vi "shooter_state_machine.vi"() -> ()   [LabVIEW 2013]
panel:
  out "Large_Cylinder_Med_Timer":i32=2000
  in  "Arm_Shooter_High":bool
  out "LAST_Shooter_Command":string
  in  "Aim":bool
  in  "Shoot":bool
  in  "Arm_Shooter_Medium":bool
  out "LAST_SHOOTER_STATE":string
  in  "Rest_Shooter":bool
  out "Large_Cylinder_CMD":bool
  out "Small_Cylinder_CMD":bool
  out "Small_Cylinder_Timer":i32=1000
  out "Large_Cylinder_High_Timer":i32=4000
  out "Shooter_Command":string
  out "Small_Cylinder_State":u8(slide) scale=0.0..1.0
  out "Large_Cylinder_State":u8(slide) scale=0.0..2.0
  out "SHOOTER_STATE":string
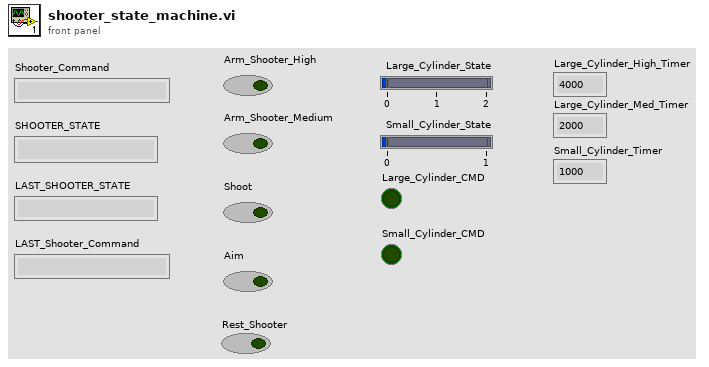
[diagram p1: front panel]
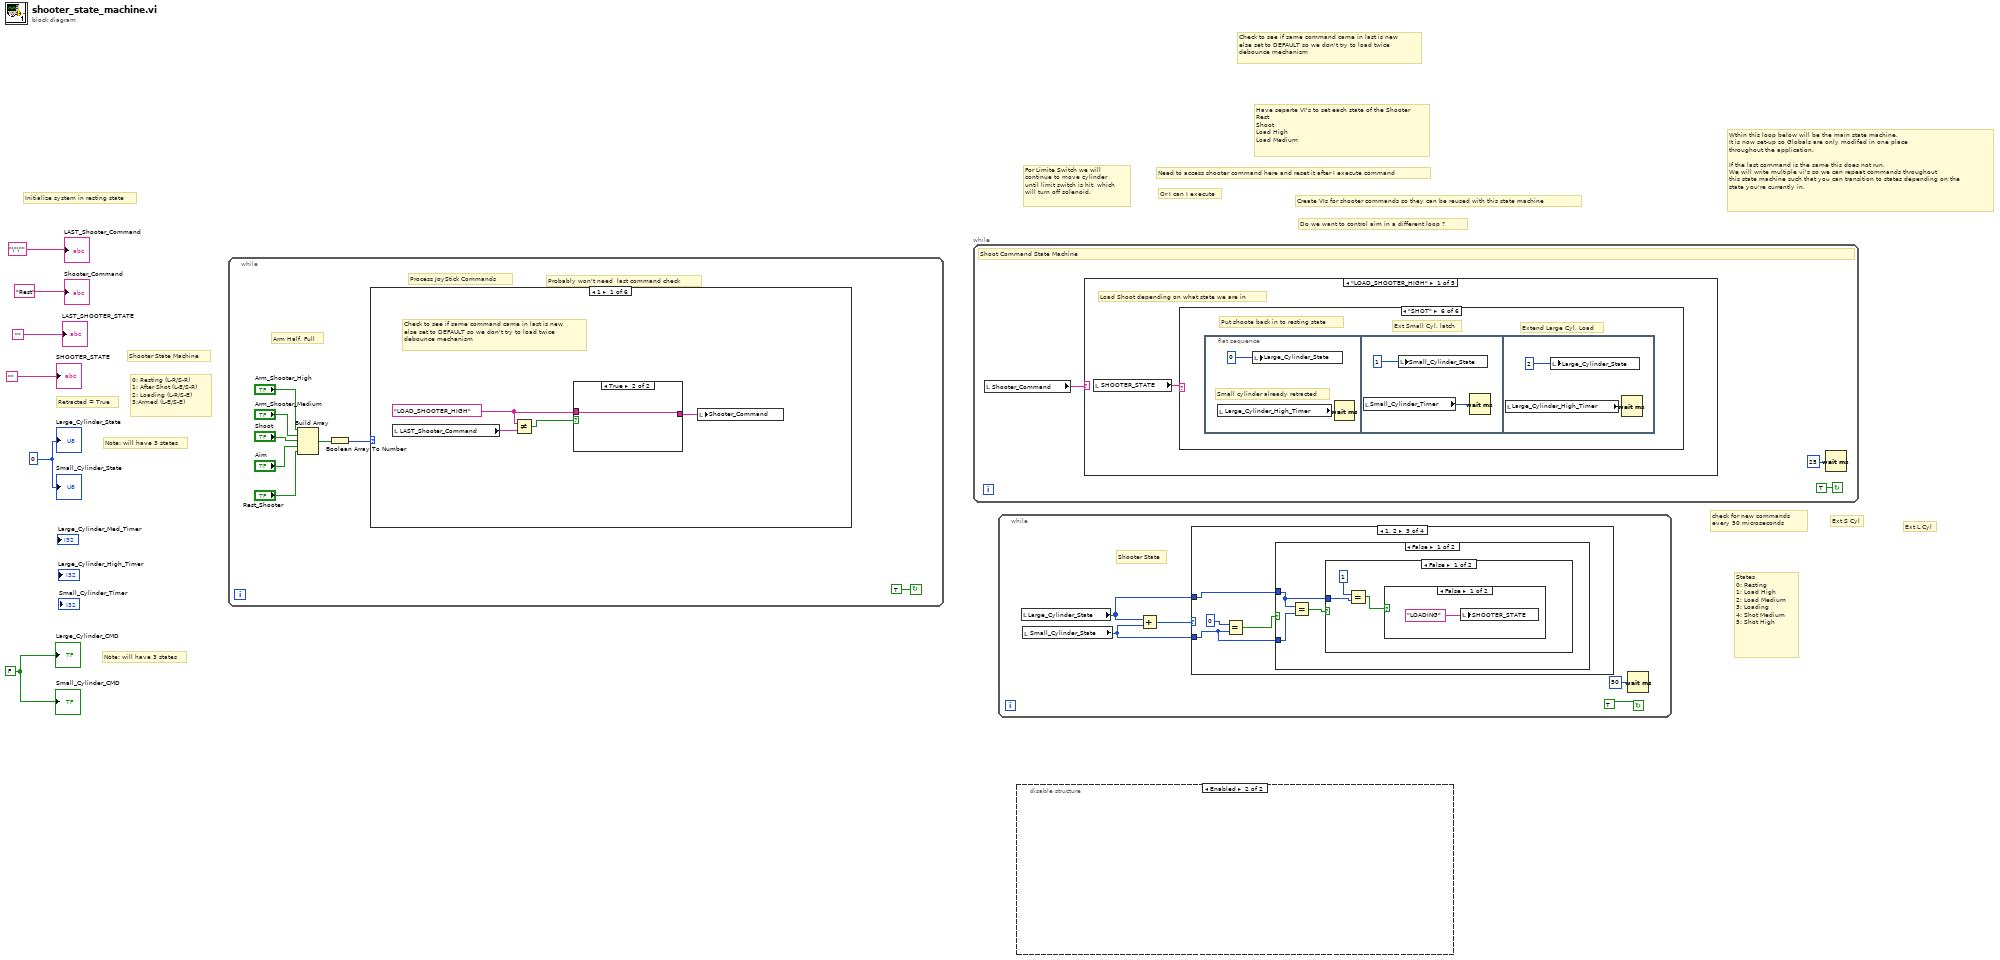
[diagram p0: block diagram]
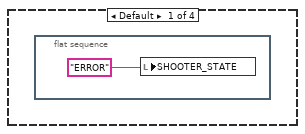
[diagram p2: hidden frame]
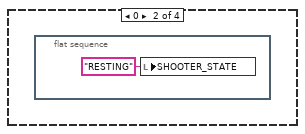
[diagram p3: hidden frame]
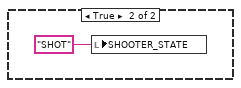
[diagram p4: hidden frame]
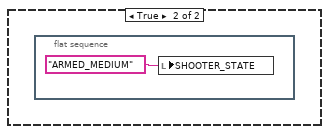
[diagram p5: hidden frame]
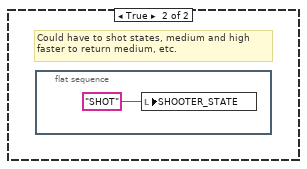
[diagram p6: hidden frame]
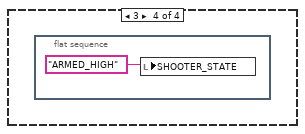
[diagram p7: hidden frame]
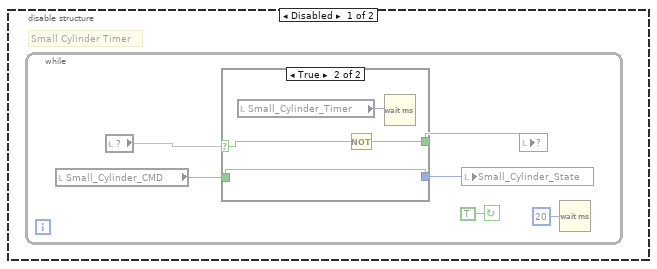
[diagram p8: hidden frame]
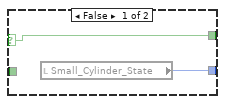
[diagram p9: hidden frame]
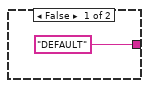
[diagram p10: hidden frame]
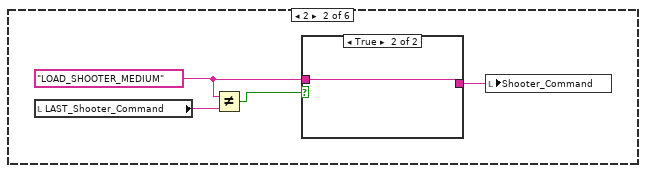
[diagram p11: hidden frame]
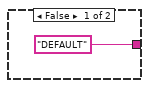
[diagram p12: hidden frame]
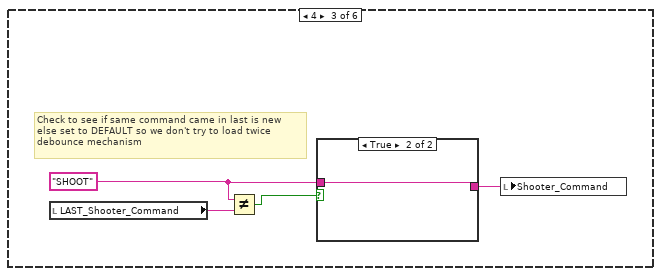
[diagram p13: hidden frame]
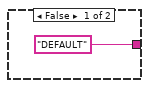
[diagram p14: hidden frame]
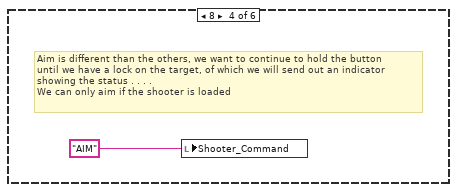
[diagram p15: hidden frame]
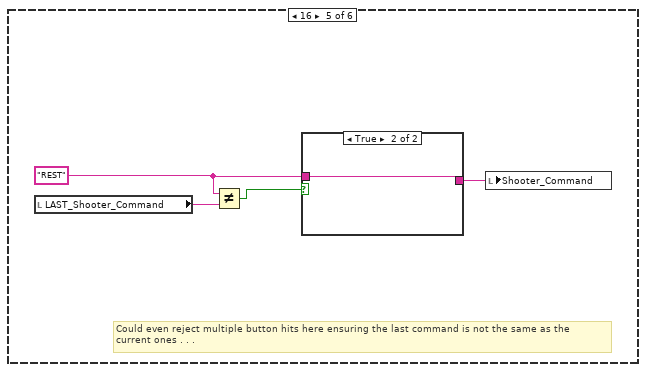
[diagram p16: hidden frame]
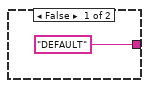
[diagram p17: hidden frame]
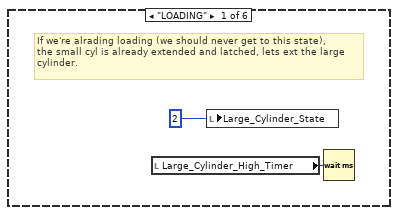
[diagram p19: hidden frame]
diagram:
  w1 = 0
  w4 = FALSE
  # "Do we want to control aim in a different loop ?"
  # "Ext L Cyl"
  # "Ext S Cyl"
  # "States\n0: Resting\n1: Load High\n2: Load Medium\n3: Loading\n4: Shot Medium\n5: Shot High"
  # "Have separte VI's to set each state of the Shooter\nRest\nShoot\nLoad High\nLoad Medium"
  # "Check to see if same command came in last is new\nelse set to DEFAULT so we don't try to load twice\ndebounce mechanism"
  # "Wthin this loop below will be the main state machine. \nIt is now set-up so Globals are only modifed in one place \nthroughout the application. \n\nIf the last command is the same this does not run.\nWe will write multiple vi's so we can repeat commands throughout\nthis state machine such that you can transition to states depending on the\nstate you're currently in."
  # "Create VIs for shooter commands so they can be reused with this state machine"
  # "check for new commands \nevery 50 microseconds"
  # "Or I can I execute"
  # "Need to access shooter command here and reset it after I execute command"
  # "Initialize system in resting state"
  # "Note: will have 3 states"
  # "0: Resting (L-R/S-R)\n1: After Shot (L-E/S-R)\n2: Loading (L-R/S-E)\n3:Armed (L-E/S-E)"
  # "For Limite Switch we will\ncontinue to move cylinder\nuntil limit switch is hit, which\nwill turn off solenoid."
  # "Note: will have 3 states"
  # "Shooter State Machine"
  # "Retracted = True"
  n1 = while {
    stop <- TRUE continue-if-true
    # "Probably won't need  last command check"
    # "Arm Half, Full"
    # "Process JoyStick Commands"
    n2 = Build Array("Arm_Shooter_High", "Arm_Shooter_Medium", "Shoot", "Aim", "Rest_Shooter") -> (w12:bool[])
    n3 = Boolean Array To Number(Boolean array=w12) -> (number=w13:u32)
    n4 = case shown="1" w13 {
      frame 1 {
        w16 = "LOAD_SHOOTER_HIGH"
        # "Check to see if same command came in last is new\nelse set to DEFAULT so we don't try to load twice\ndebounce mechanism"
        n5 = local read "LAST_Shooter_Command"() -> (w18:string)
        n6 = Not Equal?(x=w16, y=w18) -> (x != y?=w17:bool)
        n7 = case shown="True" w17 {
          tunnel: w16 -> [_ w20]
          tunnel: ["DEFAULT" w20] -> w15
          frame False {
          }
          frame True {
          }
        }
        n8 = local write "Shooter_Command"(w15) -> ()
      }
      frame 2 {
        w22 = "LOAD_SHOOTER_MEDIUM"
        n9 = local read "LAST_Shooter_Command"() -> (w24:string)
        n10 = Not Equal?(x=w22, y=w24) -> (x != y?=w23:bool)
        n11 = case shown="True" w23 {
          tunnel: w22 -> [_ w26]
          tunnel: ["DEFAULT" w26] -> w21
          frame False {
          }
          frame True {
          }
        }
        n12 = local write "Shooter_Command"(w21) -> ()
      }
      frame 4 {
        w28 = "SHOOT"
        # "Check to see if same command came in last is new\nelse set to DEFAULT so we don't try to load twice\ndebounce mechanism"
        n13 = local read "LAST_Shooter_Command"() -> (w30:string)
        n14 = Not Equal?(x=w28, y=w30) -> (x != y?=w29:bool)
        n15 = case shown="True" w29 {
          tunnel: w28 -> [_ w32]
          tunnel: ["DEFAULT" w32] -> w27
          frame False {
          }
          frame True {
          }
        }
        n16 = local write "Shooter_Command"(w27) -> ()
      }
      frame 8 {
        # "Aim is different than the others, we want to continue to hold the button\nuntil we have a lock on the target, of which we will send out an indicator \nshowing the status . . . . \nWe can only aim if the shooter is loaded"
        n17 = local write "Shooter_Command"("AIM") -> ()
      }
      frame 16 {
        w35 = "REST"
        # "Could even reject multiple button hits here ensuring the last command is not the same as the \ncurrent ones . . ."
        n18 = local read "LAST_Shooter_Command"() -> (w37:string)
        n19 = Not Equal?(x=w35, y=w37) -> (x != y?=w36:bool)
        n20 = case shown="True" w36 {
          tunnel: w35 -> [_ w39]
          tunnel: ["DEFAULT" w39] -> w34
          frame False {
          }
          frame True {
          }
        }
        n21 = local write "Shooter_Command"(w34) -> ()
      }
      frame Default {
        # "Do Nothing"
      }
    }
  }
  n22 = while "Shoot Command State Machine" {
    stop <- TRUE continue-if-true
    # "Shoot Command State Machine"
    n23 = local read "Shooter_Command"() -> (w40:string)
    n24 = case shown="\"LOAD_SHOOTER_HIGH\"" w40 {
      frame "LOAD_SHOOTER_HIGH" {
        # "Load Shoot depending on what state we are in"
        n25 = local read "SHOOTER_STATE"() -> (w43:string)
        n26 = case shown="\"SHOT\"" w43 {
          frame "LOADING" {
            # "If we're alrading loading (we should never get to this state), \nthe small cyl is already extended and latched, lets ext the large\ncylinder."
            n27 = local read "Large_Cylinder_High_Timer"() -> (w44:i32)
            n28 = local write "Large_Cylinder_State"(2) -> ()
            n29 = Wait (ms)(milliseconds to wait=w44) -> ()  [unwired: 1 out]
          }
          frame Default {
            # "Some kind of error state, should never find ourselves here"
          }
          frame "RESTING" {
            # "Ext L Cyl"
            # "Ext S Cyl"
            n30 = flat-sequence {
              frame #0 {
                n31 = local read "Small_Cylinder_Timer"() -> (w47:i32)
                n32 = local write "Small_Cylinder_State"(1) -> ()
                n33 = Wait (ms)(milliseconds to wait=w47) -> ()  [unwired: 1 out]
              }
              frame #1 {
                n34 = local read "Large_Cylinder_High_Timer"() -> (w48:i32)
                n35 = local write "Large_Cylinder_State"(2) -> ()
                n36 = Wait (ms)(milliseconds to wait=w48) -> ()  [unwired: 1 out]
              }
            }
          }
          frame "ARMED_MEDIUM" {
            # "Just need extend for half time"
            n37 = local write "Large_Cylinder_State"(2) -> ()
            n38 = local read "Large_Cylinder_Med_Timer"() -> (w50:i32)
            n39 = Wait (ms)(milliseconds to wait=w50) -> ()  [unwired: 1 out]
          }
          frame "ARMED_HIGH" {
            # "Nothing To Do Already There"
          }
          frame "SHOT" {
            # "Extend Large Cyl, Load"
            # "Ext Small Cyl, latch"
            # "Put shoote back in to resting state"
            n40 = flat-sequence {
              frame #0 {
                # "Small cylinder already retracted"
                n41 = local read "Large_Cylinder_High_Timer"() -> (w52:i32)
                n42 = local write "Large_Cylinder_State"(0) -> ()
                n43 = Wait (ms)(milliseconds to wait=w52) -> ()  [unwired: 1 out]
              }
              frame #1 {
                n44 = local read "Small_Cylinder_Timer"() -> (w55:i32)
                n45 = local write "Small_Cylinder_State"(1) -> ()
                n46 = Wait (ms)(milliseconds to wait=w55) -> ()  [unwired: 1 out]
              }
              frame #2 {
                n47 = local read "Large_Cylinder_High_Timer"() -> (w56:i32)
                n48 = local write "Large_Cylinder_State"(2) -> ()
                n49 = Wait (ms)(milliseconds to wait=w56) -> ()  [unwired: 1 out]
              }
            }
          }
        }
      }
      frame "LOAD_SHOOTER_MEDIUM" {
        # "Load Shoot depending on what state we are in"
        n50 = local read "SHOOTER_STATE"() -> (w58:string)
        n51 = case shown="\"RESTING\"" w58 {
          frame "LOADING" {
            # "If we're alrading loading (we should never get to this state), \nthe small cyl is already extended and latched, lets ext the large\ncylinder."
            n52 = local read "Large_Cylinder_Med_Timer"() -> (w59:i32)
            n53 = local write "Large_Cylinder_State"(1) -> ()
            n54 = Wait (ms)(milliseconds to wait=w59) -> ()  [unwired: 1 out]
          }
          frame Default {
            # "Some kind of error state, should never find ourselves here"
          }
          frame "RESTING" {
            # "Ext L Cyl"
            # "Ext S Cyl"
            n55 = flat-sequence {
              frame #0 {
                n56 = local read "Small_Cylinder_Timer"() -> (w62:i32)
                n57 = local write "Small_Cylinder_State"(1) -> ()
                n58 = Wait (ms)(milliseconds to wait=w62) -> ()  [unwired: 1 out]
              }
              frame #1 {
                n59 = local read "Large_Cylinder_Med_Timer"() -> (w63:i32)
                n60 = local write "Large_Cylinder_State"(1) -> ()
                n61 = Wait (ms)(milliseconds to wait=w63) -> ()  [unwired: 1 out]
              }
            }
          }
          frame "ARMED_HIGH" {
            n62 = local write "Large_Cylinder_State"(1) -> ()
            n63 = local read "Large_Cylinder_Med_Timer"() -> (w65:i32)
            n64 = Wait (ms)(milliseconds to wait=w65) -> ()  [unwired: 1 out]
          }
          frame "ARMED_MEDIUM" {
            # "Nothing To Do Already There"
          }
          frame "SHOT" {
            # "Extend Large Cyl, Load"
            # "Ext Small Cyl, latch"
            # "Put shoote back in to resting state"
            n65 = flat-sequence {
              frame #0 {
                # "Small cylinder already retracted"
                n66 = local read "Large_Cylinder_Med_Timer"() -> (w67:i32)
                n67 = local write "Large_Cylinder_State"(0) -> ()
                n68 = Wait (ms)(milliseconds to wait=w67) -> ()  [unwired: 1 out]
              }
              frame #1 {
                n69 = local read "Small_Cylinder_Timer"() -> (w70:i32)
                n70 = local write "Small_Cylinder_State"(1) -> ()
                n71 = Wait (ms)(milliseconds to wait=w70) -> ()  [unwired: 1 out]
              }
              frame #2 {
                n72 = local read "Large_Cylinder_Med_Timer"() -> (w71:i32)
                n73 = local write "Large_Cylinder_State"(1) -> ()
                n74 = Wait (ms)(milliseconds to wait=w71) -> ()  [unwired: 1 out]
              }
            }
          }
        }
      }
      frame Default {
        # "Do Nothing"
      }
      frame "REST" {
        n75 = local read "SHOOTER_STATE"() -> (w73:string)
        n76 = case shown="Default" w73 {
          frame "RESTING" {
            # "Do nothing already resting"
          }
          frame Default {
            n77 = local read "Large_Cylinder_High_Timer"() -> (w75:i32)
            n78 = local write "Large_Cylinder_State"(0) -> ()
            n79 = local write "Small_Cylinder_State"(0) -> ()
            n80 = Wait (ms)(milliseconds to wait=w75) -> ()  [unwired: 1 out]
          }
        }
      }
      frame "SHOOT" {
        # "We can only shoot\nif we are armed"
        n81 = local read "SHOOTER_STATE"() -> (w77:string)
        n82 = case shown="\"ARMED_HIGH\", \"ARMED_MEDIUM\"" w77 {
          frame Default {
            # "Do nothing"
          }
          frame "ARMED_HIGH", "ARMED_MEDIUM" {
            # "Will need to turn off at end"
            n83 = local read "Small_Cylinder_Timer"() -> (w79:i32)
            n84 = local write "Small_Cylinder_State"(0) -> ()
            n85 = Wait (ms)(milliseconds to wait=w79) -> ()  [unwired: 1 out]
          }
        }
      }
    }
    n86 = Wait (ms)(milliseconds to wait=u32 25) -> ()  [unwired: 1 out]
  }
  n87 = while {
    stop <- TRUE continue-if-true
    # "Shooter State"
    n88 = local read "Large_Cylinder_State"() -> (w81:u8)
    n89 = local read "Small_Cylinder_State"() -> (w80:u8)
    n90 = Add(x=w81, y=w80) -> (x+y=w82:u8)
    n91 = case shown="1, 2" w82 {
      tunnel: w81 -> [_ _ w88 _]
      tunnel: w80 -> [_ _ w87 _]
      frame Default {
        n92 = flat-sequence {
          frame #0 {
            n93 = local write "SHOOTER_STATE"("ERROR") -> ()
          }
        }
      }
      frame 0 {
        n94 = flat-sequence {
          frame #0 {
            n95 = local write "SHOOTER_STATE"("RESTING") -> ()
          }
        }
      }
      frame 1, 2 {
        n96 = Equal?(x=0, y=w87) -> (x = y?=w89:bool)
        n97 = case shown="False" w89 {
          tunnel: w88 -> [w91 _]
          tunnel: w87 -> [w93 _]
          frame False {
            n98 = Equal?(x=w91, y=w93) -> (x = y?=w92:bool)
            n99 = case shown="False" w92 {
              tunnel: w91 -> [w94 _]
              frame False {
                n100 = Equal?(x=1, y=w94) -> (x = y?=w96:bool)
                n101 = case shown="False" w96 {
                  frame False {
                    n102 = local write "SHOOTER_STATE"("LOADING") -> ()
                  }
                  frame True {
                    n103 = local write "SHOOTER_STATE"("SHOT") -> ()
                  }
                }
              }
              frame True {
                n104 = flat-sequence {
                  frame #0 {
                    n105 = local write "SHOOTER_STATE"("ARMED_MEDIUM") -> ()
                  }
                }
              }
            }
          }
          frame True {
            # "Could have to shot states, medium and high\nfaster to return medium, etc."
            n106 = flat-sequence {
              frame #0 {
                n107 = local write "SHOOTER_STATE"("SHOT") -> ()
              }
            }
          }
        }
      }
      frame 3 {
        n108 = flat-sequence {
          frame #0 {
            n109 = local write "SHOOTER_STATE"("ARMED_HIGH") -> ()
          }
        }
      }
    }
    n110 = Wait (ms)(milliseconds to wait=u32 50) -> ()  [unwired: 1 out]
  }
  n111 = disable-structure shown="Enabled" {
    frame Disabled {
      # "Small Cylinder Timer"
      n112 = while {
        stop <- TRUE continue-if-true
        n113 = local read "Small_Cylinder_CMD"() -> (w105:bool)
        n114 = local read item#-1() -> (w106)
        n115 = case shown="True" w106 {
          selector: w106 -> [w109 w112]
          tunnel: w105 -> [_ w110]
          tunnel: [w108 w110] -> w104
          tunnel: [w109 w111] -> w103
          frame False {
            n116 = local read "Small_Cylinder_State"() -> (w108:u8)
          }
          frame True {
            n117 = local read "Small_Cylinder_Timer"() -> (w113:i32)
            n118 = Not(x=w112) -> (.not. x?=w111:bool)
            n119 = Wait (ms)(milliseconds to wait=w113) -> ()  [unwired: 1 out]
          }
        }
        n120 = local write "Small_Cylinder_State"(w104) -> ()
        n121 = local write item#-1(w103) -> ()
        n122 = Wait (ms)(milliseconds to wait=u32 20) -> ()  [unwired: 1 out]
      }
    }
    frame Enabled {
    }
  }
  "SHOOTER_STATE" <- ""
  "Large_Cylinder_State" <- w1
  "Small_Cylinder_State" <- w1
  "Shooter_Command" <- "Rest"
  "Large_Cylinder_CMD" <- w4
  "Small_Cylinder_CMD" <- w4
  "LAST_SHOOTER_STATE" <- ""
  "LAST_Shooter_Command" <- "\"\""
